vi "Check Initial Version.vi"(0 "Build Version In":T1) -> (4 "Build Version Out":T1)   [LabVIEW 2021, in "Packager Helpers.lvlib"]
uses:
  <vilib>/AppBuilder/AB_API_Simple/Build Specification Version.ctl
  Packager Helpers.lvlib
  <vilib>/AppBuilder/AB_API_Simple/NI_App_Builder_API.lvlib
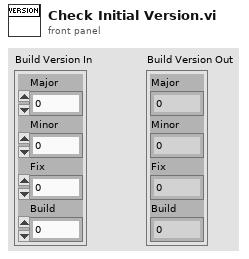
[diagram p1: front panel]
types:
  T1 = typedef "NI_App_Builder_API.lvlib/Build Specification Version.ctl" = cluster{"Major":u16, "Minor":u16, "Fix":u16, "Build":u16}
  T2 = cluster{"Major":bool, "Minor":bool, "Fix":bool, "Build":bool}
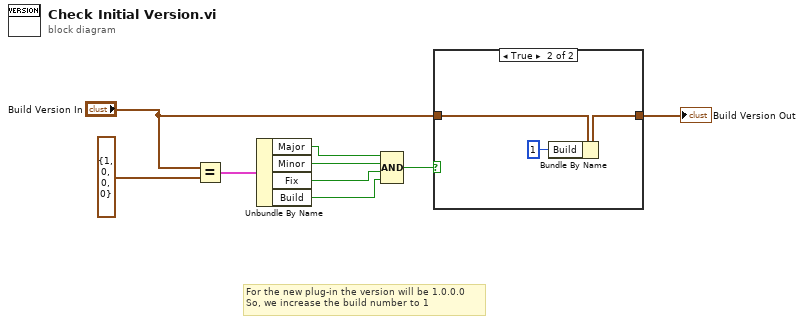
[diagram p0: block diagram]
diagram:
  # "For the new plug-in the version will be 1.0.0.0\nSo, we increase the build number to 1"
  n1 = Equal?(x="Build Version In", y=T1 {"Major"=1, "Minor"=0, "Fix"=0, "Build"=0}) -> (x = y?=w8:T2)
  n2 = Unbundle By Name(w8) -> ("Major"=w7:bool, "Minor"=w6:bool, "Fix"=w5:bool, "Build"=w4:bool)
  n3 = Compound Arithmetic op=AND(w7, w6, w5, w4) -> (w3:bool)
  n4 = case shown="True" w3 {
    tunnel: "Build Version In" -> [w10 w13]
    tunnel: [w10 w11] -> w1
    frame False {
    }
    frame True {
      n5 = Bundle By Name(cluster=w13, "Build"=u16 1) -> (w11:T1)
    }
  }
  "Build Version Out" <- w1
